vi "Handle Last Ack Core.vi"(4 "Error In":errorcluster, 6 "Last Ack":refnum<class "Last Ack.lvclass">, 7 "LHW-GUI-Actor in":refnum<class "LHW-GUI-Actor.lvclass">) -> (0 "Error Out":errorcluster, 3 "LHW-GUI-Actor out":refnum<class "LHW-GUI-Actor.lvclass">)   [LabVIEW 2014, in "LHW-GUI.lvlib" / "LHW-GUI-Actor.lvclass"]
doc: "(<B>Filename</B>: Actor Framework.lvlib:Actor.lvclass:Handle Last Ack Core.vi)\n\nDefines how the caller actor responds to the Last Ack message from a nested actor. The Last Ack message is the final message a nested actor sends to its caller before it shuts down. The message contains information about the final state of the nested actor.\n\nBy default, this method does nothing except return any error the nested actor sent. A descendant class may override this method to define behavior."
uses:
  LHW-GUI-Actor.lvclass
  <vilib>/ActorFramework/LastAck/Last Ack.lvclass
  LHW-GUI-Actor.lvclass/LHW-GUI-Actor.ctl
  <vilib>/ActorFramework/LastAck/Last Ack.lvclass/Last Ack.ctl
  <vilib>/ActorFramework/Actor/Actor.lvclass
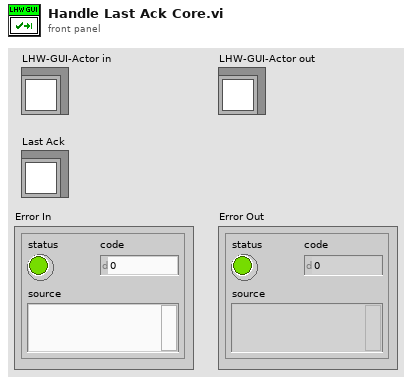
[diagram p1: front panel]
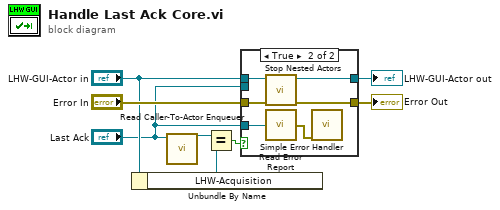
[diagram p0: block diagram]
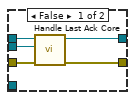
[diagram p2: hidden frame]
diagram:
  n1 = Unbundle By Name("LHW-GUI-Actor in") -> ("LHW-Acquisition"=w4:refnum<class "Message Enqueuer.lvclass">)
  n2 = call <vilib>:"Read Caller-To-Actor Enqueuer.vi"("Last Ack"="Last Ack") -> ("Caller-to-Actor Enqueuer"=w3:refnum<class "Message Enqueuer.lvclass">)  [unwired: 10 in]
  n3 = Equal?(x=w3, y=w4) -> (x = y?=w2:bool)
  n4 = case shown="True" w2 {
    tunnel: [w13 w16] -> w8
    tunnel: [w12 w18] -> w7
    tunnel: "Error In" -> [w11 w17]
    tunnel: "Last Ack" -> [w10 _]
    tunnel: "LHW-GUI-Actor in" -> [w9 w19]
    tunnel: "Last Ack" -> [_ w15]
    frame False {
      n5 = call-parent "Handle Last Ack Core.vi"("error in (no error)"=w11, "Last Ack"=w10, "Actor in"=w9) -> ("error out"=w13:errorcluster, "Actor out"=w12:refnum<class "LHW-GUI-Actor.lvclass">)  [unwired: 3 in]
    }
    frame True {
      n6 = call "Stop Nested Actors.vi"("Error In"=w17, "LHW-GUI-Actor in"=w19) -> ("Error Out"=w16:errorcluster, "LHW-GUI-Actor out"=w18:refnum<class "LHW-GUI-Actor.lvclass">)  [unwired: 8 in]
      n7 = call <vilib>:"Read Error Report.vi"("Last Ack"=w15) -> ("error report"=w14:errorcluster)
      n8 = call <vilib>:"Simple Error Handler.vi"("error in (no error)"=w14) -> ()  [unwired: 4 in, 5 out]
    }
  }
  "LHW-GUI-Actor out" <- w7
  "Error Out" <- w8
